vi "NameData_Variant Scalar to String Value.vi"(5 "Format Cluster":T1, 7 "String Format Select":T2, 8 "Error":errorcluster, 11 "Variant":variant) -> (0 "Error Out":errorcluster, 2 "Name Out":string, 3 "Value Out":string)   [LabVIEW 2020]
uses:
  TypeDefs_Utility/ENUM_NameData_String Format Select.ctl
  TypeDefs_Utility/Cluster_NameData_String Format Data.ctl
  <vilib>/Utility/VariantDataType/VariantType.lvlib
  <vilib>/Utility/Data Type/NI_Data Type.lvlib
panel:
  # "%.2f %g %e %p"
  # "%d %h %o %b"
  # "'%s'"
  # "%x %X"
  # "True,False -1,0 Yes,No"
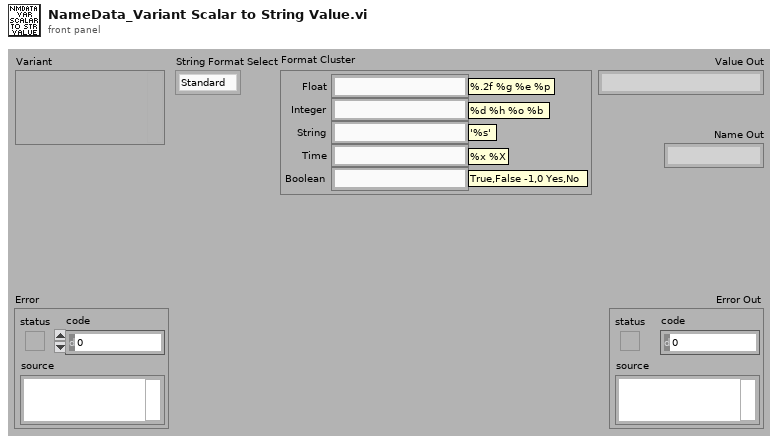
[diagram p1: front panel]
types:
  T1 = typedef "Cluster_NameData_String Format Data.ctl" = cluster{"Float":string, "Integer":string, "String":string, "Time":string, "Boolean":string}
  T2 = typedef "ENUM_NameData_String Format Select.ctl" = enum16{"Standard", "Access DB", "Custom"}
  T3 = typedef "NI_Data Type.lvlib/Data Type.ctl" = enum8{"Invalid Type", "Void", "I8", "I16", "I32", "I64", "U8", "U16", "U32", "U64", "Single Float", "Double Float", "Extended Float", "Single Complex", "Double Complex", "Extended Complex", "Enum U8", "Enum U16", "Enum U32", "Enum U64", "Single Float With Unit", "Double Float With Unit", "Extended Float With Unit", "Single Complex with Unit", "Double Complex with Unit", "Extended Complex with Unit", "Boolean", "String", "Path", "Picture", "Tag", "Array", "Cluster", "Variant", "LV Variant", "Waveform", "Timestamp", "Digital Waveform", "Digital Data", "ExpressData", "Refnum", "External Data", "VI", "Poly VI", "LabVIEW Class Instance", "Fixed Point", "Set Collection", "Map Collection"}
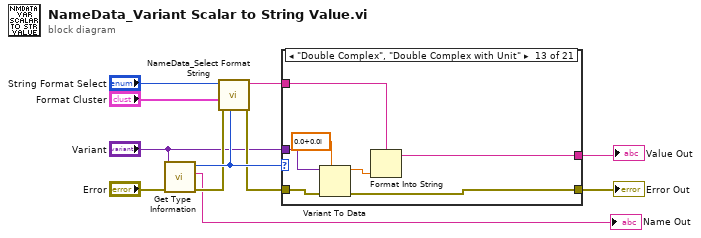
[diagram p0: block diagram]
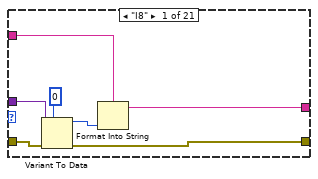
[diagram p2: hidden frame]
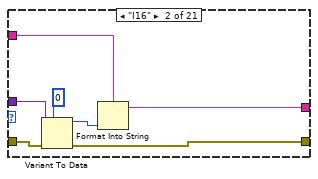
[diagram p3: hidden frame]
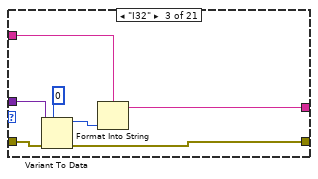
[diagram p4: hidden frame]
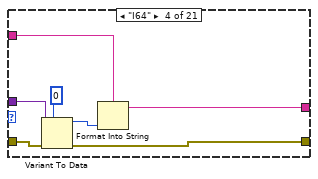
[diagram p5: hidden frame]
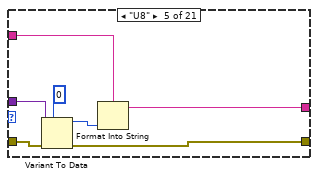
[diagram p6: hidden frame]
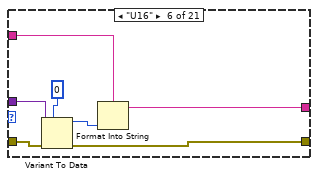
[diagram p7: hidden frame]
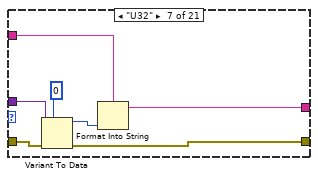
[diagram p8: hidden frame]
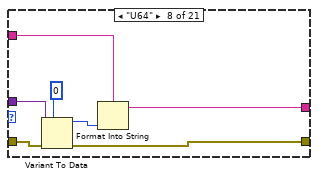
[diagram p9: hidden frame]
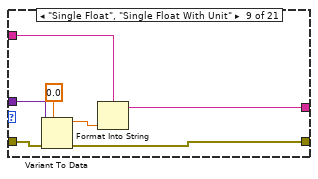
[diagram p10: hidden frame]
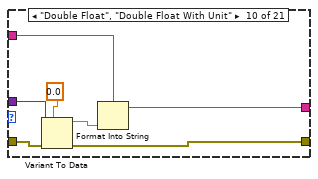
[diagram p11: hidden frame]
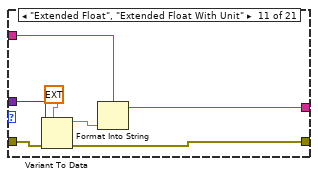
[diagram p12: hidden frame]
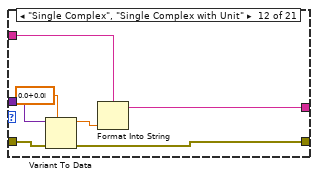
[diagram p13: hidden frame]
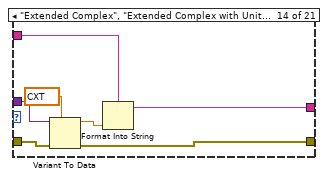
[diagram p14: hidden frame]
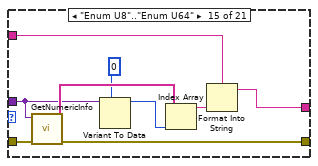
[diagram p15: hidden frame]
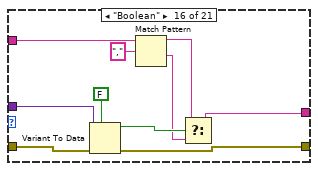
[diagram p16: hidden frame]
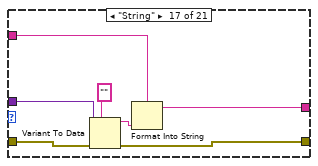
[diagram p17: hidden frame]
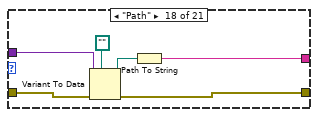
[diagram p18: hidden frame]
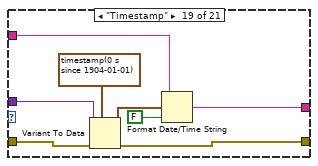
[diagram p19: hidden frame]
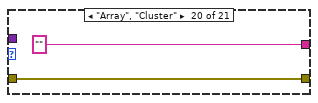
[diagram p20: hidden frame]
diagram:
  n1 = call <vilib>:"Get Type Information.vi"("error in (no error)"="Error", "variant"="Variant") -> ("error out"=w6:errorcluster, "name"=→"Name Out":string, "type"=w11:T3)  [unwired: 5 in, 2 out]
  n2 = call "NameData_Select Format String.vi"("Data Type"=w11, "Error"=w6, "Format Cluster"="Format Cluster", "String Format Select"="String Format Select") -> ("Error Out"=w7:errorcluster, "Format String Out"=w8:string)  [unwired: 6 in]
  n3 = case shown="\"Double Complex\", \"Double Complex with Unit\"" w11 {
    tunnel: [w15 w22 w29 w36 w43 w50 w57 w64 w71 w78 w85 w92 w99 w106 w113 w128 w135 w141 w149 w151 w159] -> w2
    tunnel: w7 -> [w18 w25 w32 w39 w46 w53 w60 w67 w74 w81 w88 w95 w102 w109 w118 w125 w132 w138 w147 w151 w159]
    tunnel: "Variant" -> [w17 w24 w31 w38 w45 w52 w59 w66 w73 w80 w87 w94 w101 w108 w116 w126 w133 w139 w148 _ w158]
    tunnel: [w13 w20 w27 w34 w41 w48 w55 w62 w69 w76 w83 w90 w97 w104 w111 w123 w129 w136 w143 "" ("Data Out") w152] -> w3
    tunnel: w8 -> [w12 w19 w26 w33 w40 w47 w54 w61 w68 w75 w82 w89 w96 w103 w110 w122 w131 _ w145 _ _]
    frame "I8" {
      n4 = Variant To Data(error in=w18, type=i8 0, Variant=w17) -> (data=w14:i8, error out=w15:errorcluster)
      n5 = Format Into String(format string=w12, w14) -> (resulting string=w13:string)  [unwired: 2 in, 1 out]
    }
    frame "I16" {
      n6 = Variant To Data(error in=w25, type=i16 0, Variant=w24) -> (data=w21:i16, error out=w22:errorcluster)
      n7 = Format Into String(format string=w19, w21) -> (resulting string=w20:string)  [unwired: 2 in, 1 out]
    }
    frame "I32" {
      n8 = Variant To Data(error in=w32, type=0, Variant=w31) -> (data=w28:i32, error out=w29:errorcluster)
      n9 = Format Into String(format string=w26, w28) -> (resulting string=w27:string)  [unwired: 2 in, 1 out]
    }
    frame "I64" {
      n10 = Variant To Data(error in=w39, type=i64 0, Variant=w38) -> (data=w35:i64, error out=w36:errorcluster)
      n11 = Format Into String(format string=w33, w35) -> (resulting string=w34:string)  [unwired: 2 in, 1 out]
    }
    frame "U8" {
      n12 = Variant To Data(error in=w46, type=u8 0, Variant=w45) -> (data=w42:u8, error out=w43:errorcluster)
      n13 = Format Into String(format string=w40, w42) -> (resulting string=w41:string)  [unwired: 2 in, 1 out]
    }
    frame "U16" {
      n14 = Variant To Data(error in=w53, type=u16 0, Variant=w52) -> (data=w49:u16, error out=w50:errorcluster)
      n15 = Format Into String(format string=w47, w49) -> (resulting string=w48:string)  [unwired: 2 in, 1 out]
    }
    frame "U32" {
      n16 = Variant To Data(error in=w60, type=u32 0, Variant=w59) -> (data=w56:u32, error out=w57:errorcluster)
      n17 = Format Into String(format string=w54, w56) -> (resulting string=w55:string)  [unwired: 2 in, 1 out]
    }
    frame "U64" {
      n18 = Variant To Data(error in=w67, type=u64 0, Variant=w66) -> (data=w63:u64, error out=w64:errorcluster)
      n19 = Format Into String(format string=w61, w63) -> (resulting string=w62:string)  [unwired: 2 in, 1 out]
    }
    frame "Single Float", "Single Float With Unit" {
      n20 = Variant To Data(error in=w74, type=sgl 0.0, Variant=w73) -> (data=w70:sgl, error out=w71:errorcluster)
      n21 = Format Into String(format string=w68, w70) -> (resulting string=w69:string)  [unwired: 2 in, 1 out]
    }
    frame "Double Float", "Double Float With Unit" {
      n22 = Variant To Data(error in=w81, type=0.0, Variant=w80) -> (data=w77:dbl, error out=w78:errorcluster)
      n23 = Format Into String(format string=w75, w77) -> (resulting string=w76:string)  [unwired: 2 in, 1 out]
    }
    frame "Extended Float", "Extended Float With Unit" {
      n24 = Variant To Data(error in=w88, type=ext 0.0, Variant=w87) -> (data=w84:ext, error out=w85:errorcluster)
      n25 = Format Into String(format string=w82, w84) -> (resulting string=w83:string)  [unwired: 2 in, 1 out]
    }
    frame "Single Complex", "Single Complex with Unit" {
      n26 = Variant To Data(error in=w95, type=csg 0.0+0.0i, Variant=w94) -> (data=w91:csg, error out=w92:errorcluster)
      n27 = Format Into String(format string=w89, w91) -> (resulting string=w90:string)  [unwired: 2 in, 1 out]
    }
    frame "Double Complex", "Double Complex with Unit" {
      n28 = Variant To Data(error in=w102, type=cdb 0.0+0.0i, Variant=w101) -> (data=w98:cdb, error out=w99:errorcluster)
      n29 = Format Into String(format string=w96, w98) -> (resulting string=w97:string)  [unwired: 2 in, 1 out]
    }
    frame "Extended Complex", "Extended Complex with Unit" {
      n30 = Variant To Data(error in=w109, type=cxt 0.0+0.0i, Variant=w108) -> (data=w105:cxt, error out=w106:errorcluster)
      n31 = Format Into String(format string=w103, w105) -> (resulting string=w104:string)  [unwired: 2 in, 1 out]
    }
    frame "Enum U8".."Enum U64" {
      n32 = call <vilib>:"GetNumericInfo.vi"("error in (no error)"=w118, "Variant"=w116) -> ("error out"=w113:errorcluster, "EnumNames"=w117:string[])  [unwired: 6 in, 2 out]
      n33 = Variant To Data(type=0, Variant=w116) -> (data=w114:i32)  [unwired: 1 in, 1 out]
      n34 = Index Array(array=w117, index=w114) -> (element=w112:string)
      n35 = Format Into String(format string=w110, w112) -> (resulting string=w111:string)  [unwired: 2 in, 1 out]
    }
    frame "Boolean" {
      n36 = Variant To Data(error in=w125, type=FALSE, Variant=w126) -> (data=w124:bool, error out=w128:errorcluster)
      n37 = Match Pattern(string=w122, regular expression=",") -> (before substring=w120:string, after substring=w119:string)  [unwired: 1 in, 2 out]
      n38 = Select(t=w120, s=w124, f=w119) -> (s? t:f=w123:string)
    }
    frame "String" {
      n39 = Variant To Data(error in=w132, type="", Variant=w133) -> (data=w130:string, error out=w135:errorcluster)
      n40 = Format Into String(format string=w131, w130) -> (resulting string=w129:string)  [unwired: 2 in, 1 out]
    }
    frame "Path" {
      n41 = Variant To Data(error in=w138, type=path "", Variant=w139) -> (data=w137:path, error out=w141:errorcluster)
      n42 = Path To String(path=w137) -> (string=w136:string)
    }
    frame "Timestamp" {
      n43 = Variant To Data(error in=w147, type=timestamp(0 s since 1904-01-01), Variant=w148) -> (data=w144:timestamp, error out=w149:errorcluster)
      n44 = Format Date/Time String(time format string (%c)=w145, seconds (now)=w144, UTC format=FALSE) -> (date/time string=w143:string)
    }
    frame "Array", "Cluster" {
    }
    frame Default {
      n45 = Variant To Flattened String(Variant=w158) -> (data string=w153:string)  [unwired: 1 out]
      n46 = String To Byte Array(string=w153) -> (unsigned byte array=w157:u8[])
      n47 = Number To Hexadecimal String(1:i16 2 ("width (-)"), 2:w157) -> (0:w156:string[])
      n48 = Concatenate Strings("0x", w156) -> (w152:string)
    }
  }
  "Value Out" <- w3
  "Error Out" <- w2
